vi "average data and create table strings.vi"(10 "Cluster in":T1={"rigChannels"=[], "rigUnits"=[], "logging"=FALSE, "chartRef"=refnum, "dataTableRef"=refnum, "channelCount"=0, "trendIndex"=0, "channels"={"massflow"=0, "PR"=0, "recircTemp"=0}, "History"={"speedlines"=[], "liveTail"={"mDot"=[], "pRatio"=[]}, "current"={"mDot"=0.0, "pRatio"=0.0}, "insertPoint"=0, "tempHistory"=[]}, "filter"=FALSE, "filterLength"=0, "tableUpdate"=0, "limitValues"=[[0.0, 45000.0], [0.0, 100.0], [0.0, 100.0], [10.0, 100.0], [0.0, 100.0], [10.0, 35.0], [0.0, 100.0], [0.0, 100.0], [99000.0, 300000.0], [-5000.0, 5000.0], [99000.0, 300000.0], [-0.01, 0.3], [-0.01, 4.5], [-0.1, 100.0], [1.0, 8.0], [1.0, 5.0], [0.0, 100.0], [0.0, 100.0], [0.0, 100.0], [-100.0, 45000.0], [-0.1, 1.0], [0.8, 2.0], [90000.0, 110000.0], [15.0, 35.0], [0.0, 0.0], [0.0, 0.0], [0.0, 0.0], [0.0, 0.0]]}, 11 "rigData":variant) -> (0 "cluster out":T1={"rigChannels"=[], "rigUnits"=[], "logging"=FALSE, "chartRef"=refnum, "dataTableRef"=refnum, "channelCount"=0, "trendIndex"=0, "channels"={"massflow"=0, "PR"=0, "recircTemp"=0}, "History"={"speedlines"=[], "liveTail"={"mDot"=[], "pRatio"=[]}, "current"={"mDot"=0.0, "pRatio"=0.0}, "insertPoint"=0, "tempHistory"=[]}, "filter"=FALSE, "filterLength"=0, "tableUpdate"=0, "limitValues"=[[0.0, 45000.0], [0.0, 100.0], [0.0, 100.0], [10.0, 100.0], [0.0, 100.0], [10.0, 35.0], [0.0, 100.0], [0.0, 100.0], [99000.0, 300000.0], [-5000.0, 5000.0], [99000.0, 300000.0], [-0.01, 0.3], [-0.01, 4.5], [-0.1, 100.0], [1.0, 8.0], [1.0, 5.0], [0.0, 100.0], [0.0, 100.0], [0.0, 100.0], [-100.0, 45000.0], [-0.1, 1.0], [0.8, 2.0], [90000.0, 110000.0], [15.0, 35.0], [0.0, 0.0], [0.0, 0.0], [0.0, 0.0], [0.0, 0.0]]}, 2 "averagedData":dbl[](array[numeric]), 3 "tableData":string[][](array[string]), 5 "updateTable":bool)   [LabVIEW 2018]
uses:
  custom sub vis/speedlineData.ctl
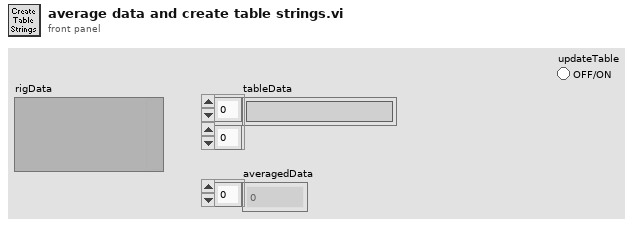
[diagram p1: front panel]
types:
  T1 = typedef "speedlineData.ctl" = cluster{"rigChannels":string[], "rigUnits":string[], "logging":bool, "chartRef":refnum<vi>, "dataTableRef":refnum<vi>, "channelCount":i32, "trendIndex":i32, "channels":cluster{"massflow":i32, "PR":i32, "recircTemp":i32}, "History":cluster{"speedlines":cluster{"mDot":dbl[], "pRatio":dbl[]}[], "liveTail":cluster{"mDot":dbl[], "pRatio":dbl[]}, "current":cluster{"mDot":dbl, "pRatio":dbl}, "insertPoint":i32, "tempHistory":dbl[][]}, "filter":bool, "filterLength":i32, "tableUpdate":i16, "limitValues":dbl[][]}
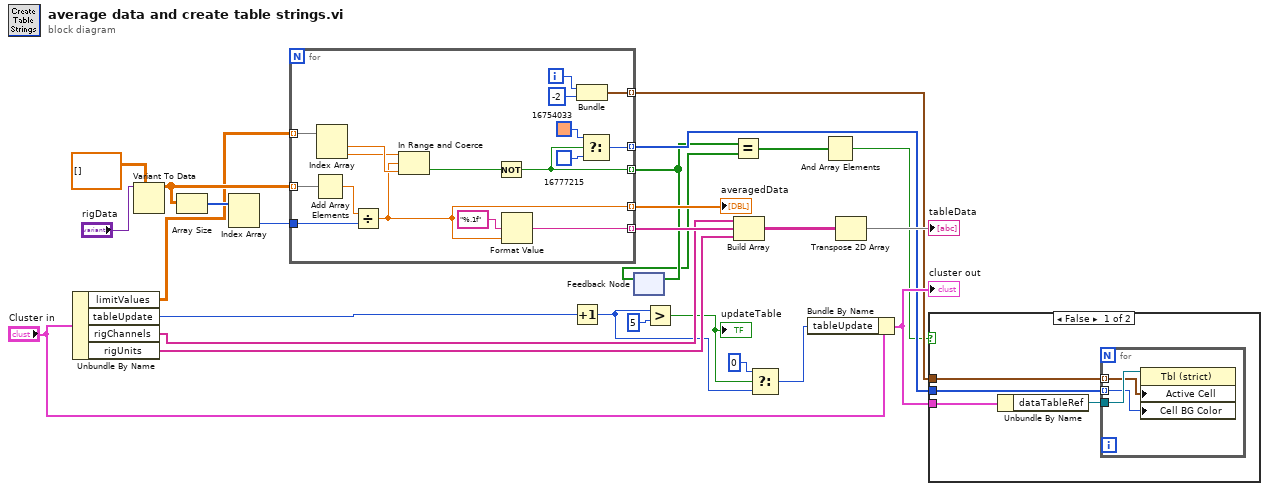
[diagram p0: block diagram]
diagram:
  n1 = Unbundle By Name("Cluster in") -> ("limitValues"=w1:dbl[][], "tableUpdate"=w11:i16, "rigChannels"=w22:string[], "rigUnits"=w23:string[])
  n2 = Variant To Data(type=dbl[][] [], Variant="rigData") -> (data=w18:dbl[][])  [unwired: 1 in, 1 out]
  n3 = Array Size(array=w18) -> (size(s)=w17:i32[])
  n4 = Index Array(array=w17) -> (element #2=w19:i32)  [unwired: 2 in, 1 out]
  n5 = for {
    tunnel: w18 -> [w43] mode=indexing
    tunnel: w19 -> [w41]
    tunnel: [w35] -> w26 mode=indexing
    tunnel: [w39] -> w24 mode=indexing
    tunnel: w1 -> [w38] mode=indexing
    tunnel: [w28] -> w5 mode=indexing
    tunnel: [w31] -> w7 mode=indexing
    tunnel: [w27] -> w6 mode=indexing
    i -> [w33]
    n6 = Add Array Elements(numeric array=w43) -> (sum=w42:dbl)
    n7 = Index Array(array=w38) -> (element #1=w37:dbl, element #2=w36:dbl)  [unwired: 2 in]
    n8 = Divide(x=w42, y=w41) -> (x/y=w35:dbl)
    n9 = In Range and Coerce(upper limit=w36, x=w35, lower limit=w37) -> (In Range?=w34:bool)  [unwired: 1 out]
    n10 = Not(x=w34) -> (.not. x?=w28:bool)
    n11 = Format Value(format string="%.1f", value (0)=w35) -> (output string=w39:string)  [unwired: 1 in]
    n12 = Bundle(w33, -2) -> (w31:cluster{i32, i32})  [unwired: 1 in]
    n13 = Select(t=u32 16754033, s=w28, f=u32 16777215) -> (s? t:f=w27:u32)
  }
  "averagedData" <- w26
  n14 = Increment(x=w11) -> (x+1=w13:i16)
  n15 = feedback-in #1(w5) -> ()
  n16 = feedback #1() -> (w4:bool[])  [unwired: 1 in]
  n17 = Greater?(x=w13, y=i16 5) -> (0:w9:bool)
  "updateTable" <- w9
  n18 = Equal?(x=w5, y=w4) -> (x = y?=w3:bool[])
  n19 = Build Array(w22, w24, w23) -> (w20:string[][])
  n20 = Select(t=i16 0, s=w9, f=w13) -> (s? t:f=w10:i16)
  n21 = Bundle By Name(cluster="Cluster in", "tableUpdate"=w10) -> (w8:T1)
  "cluster out" <- w8
  n22 = And Array Elements(Boolean array=w3) -> (logical AND=w2:bool)
  n23 = Transpose 2D Array(2D array=w20) -> (transposed array=→"tableData":string[][])
  n24 = case shown="False" w2 {
    tunnel: w8 -> [w47 _]
    tunnel: w7 -> [w45 _]
    tunnel: w6 -> [w44 _]
    frame False {
      n25 = Unbundle By Name(w47) -> ("dataTableRef"=w46:refnum<vi>)
      n26 = for {
        tunnel: w46 -> [w50]
        tunnel: w45 -> [w49] mode=indexing
        tunnel: w44 -> [w48] mode=indexing
        n27 = property class="Tbl (strict)"(reference=w50, "Active Cell"=w49, "Cell BG Color"=w48) -> ()  [unwired: 1 in, 2 out]
      }
    }
    frame True {
    }
  }
